vi "Self-Test.vi"(8 "error in (no error)":errorcluster, 11 "VISA resource name":refnum<visa-resource-name>) -> (0 "error out":errorcluster, 1 "Self-Test Result Message":string, 2 "Self-Test Result Code":i32, 3 "VISA resource name out":refnum<visa-resource-name>)   [LabVIEW 2020, in "MagnaDC.lvlib"]
doc: "Runs the instrument's self-test routine and returns the test results."
uses:
  MagnaDC.lvlib
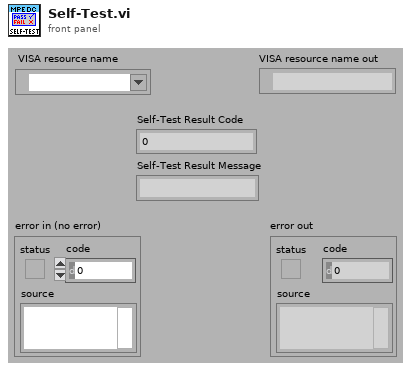
[diagram p1: front panel]
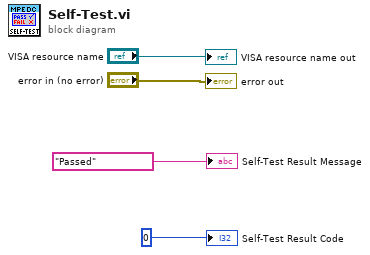
[diagram p0: block diagram]
diagram:
  "Self-Test Result Message" <- "Passed"
  "Self-Test Result Code" <- 0
  "VISA resource name out" <- "VISA resource name"
  "error out" <- "error in (no error)"
